vi "Get Devices.vi"(8 "error in (no error)":errorcluster, 11 "DeviceListPanel in":refnum<class "DeviceListPanel.lvclass">) -> (0 "error out":errorcluster, 2 "Devices":refnum<class "Device.lvclass">[](array[class]), 3 "DeviceListPanel out":refnum<class "DeviceListPanel.lvclass">)   [LabVIEW 2020, in "PicoG-App.lvlib" / "DeviceListPanel.lvclass"]
uses:
  DeviceListPanel.lvclass
  Device/Device.lvclass
  DeviceListPanel.lvclass/DeviceListPanel.ctl
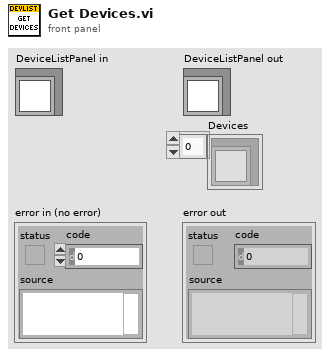
[diagram p1: front panel]
types:
  T1 = typedef "PicoG-App.lvlib/DeviceListPanel.lvclass/Ref Data.ctl" = cluster{"Map":map{T2, T3}}
  T2 = typedef "PicoG-App.lvlib/Device.lvclass/Device Key.ctl" = cluster{"Platform":string, "Board":string, "ID":string}
  T3 = typedef "PicoG-App.lvlib/DeviceListPanel.lvclass/Device and Panel.ctl" = cluster{"Device":refnum<class "Device.lvclass">, "Panel":refnum<class "DeviceArrayPanel.lvclass">}
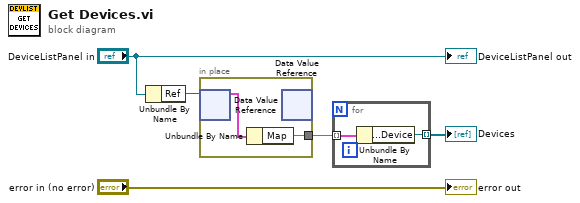
[diagram p0: block diagram]
diagram:
  n1 = Unbundle By Name("DeviceListPanel in") -> ("Ref"=w4:refnum<data-value>)
  n2 = in-place {
    in-place-border: [w6] -> w2
    n3 = in-place-dvr #1(w4) -> (w7:T1)  [unwired: 1 out]
    n4 = Unbundle By Name(w7) -> ("Map"=w6:map{T2, T3})
    n5 = in-place-dvr #1() -> ()  [unwired: 1 in, 2 out]
  }
  n6 = for {
    tunnel: w2 -> [w9] mode=indexing
    tunnel: [w8] -> w1 mode=indexing
    n7 = Unbundle By Name(w9) -> ("Value Type.Device"=w8:refnum<class "Device.lvclass">)
  }
  "Devices" <- w1
  "error out" <- "error in (no error)"
  "DeviceListPanel out" <- "DeviceListPanel in"
